vi "Write Message Channel Type.vi"(8 "error in (no error)":errorcluster, 10 "Message Channel Type":refnum<class "Pub Sub Message Channel.lvclass">, 11 "Simple Chat in":refnum<class "Simple Chat.lvclass">) -> (0 "error out":errorcluster, 3 "Simple Chat out":refnum<class "Simple Chat.lvclass">)   [LabVIEW 2020, in "Simple Chat.lvlib" / "Simple Chat.lvclass"]
uses:
  Simple Chat.lvclass
  Actor Pub Sub Channels/Pub Sub Message Channel/Pub Sub Message Channel.lvclass
  Simple Chat.lvclass/Simple Chat.ctl
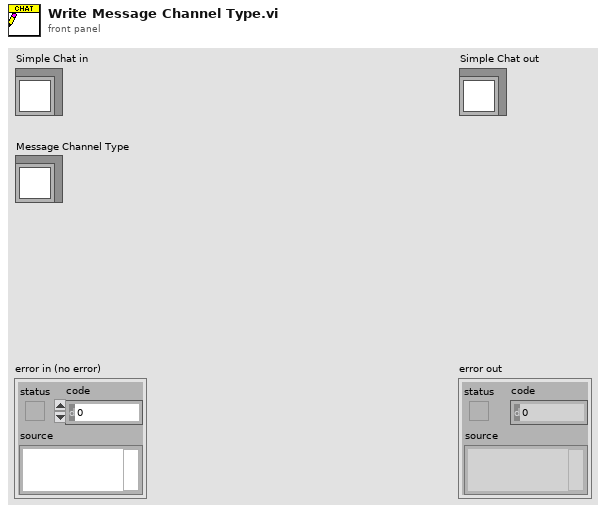
[diagram p1: front panel]
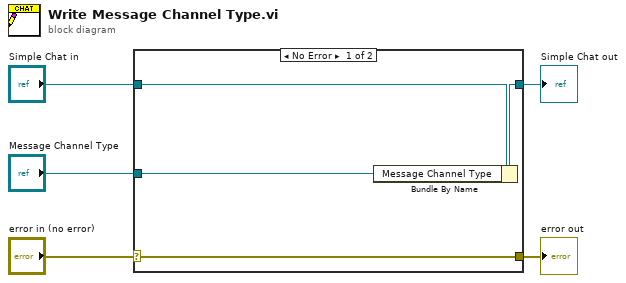
[diagram p0: block diagram]
diagram:
  n1 = case shown="No Error" "error in (no error)" {
    selector: "error in (no error)" -> [w9 w10]
    tunnel: [w9 w10] -> w4
    tunnel: [w7 w11] -> w2
    tunnel: "Simple Chat in" -> [w8 w11]
    tunnel: "Message Channel Type" -> [w6 _]
    frame No Error {
      n2 = Bundle By Name(cluster=w8, "Message Channel Type"=w6) -> (w7:refnum<class "Simple Chat.lvclass">)
    }
    frame Error {
    }
  }
  "error out" <- w4
  "Simple Chat out" <- w2
